vi "Write_Bypass.vi"(0 "AccelNET.lvlib:TCP.lvclass":refnum<class "TCP.lvclass">, 2 "Pelletron Bypass":T1, 3 "error in (no error)":errorcluster) -> (10 "Error Out":errorcluster)   [LabVIEW 2012, in "AccelNET.lvlib" / "TCP.lvclass"]
uses:
  TCP.lvclass
  Bypass_Control.ctl
  Useful_SubVIs.lvlib
  Useful_Controls.lvlib
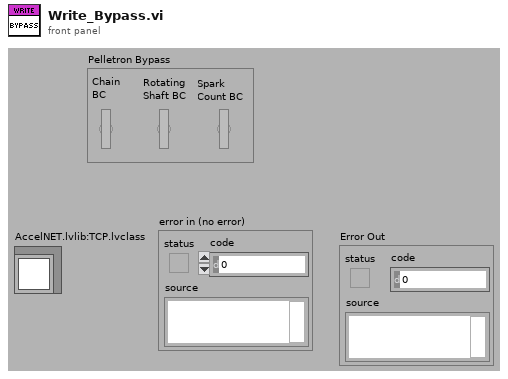
[diagram p1: front panel]
types:
  T1 = typedef "AccelNET.lvlib/Useful_Controls.lvlib/Bypass_Control.ctl" = cluster{"Chain\nBC":bool, "Rotating\nShaft BC":bool, "Spark\nCount BC":bool}
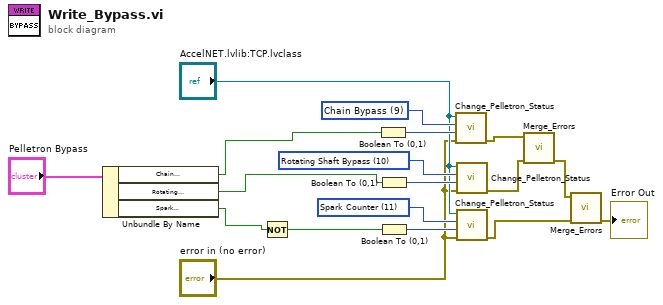
[diagram p0: block diagram]
diagram:
  w14 = u16 11 items=["GV", "Blower", "Main Power Supply", "Chain Power Supply", "Chain", "Rotating Shaft", "Power Supply Voltage", "Control Mode", "Control Mode Reference", "Chain Bypass", "Rotating Shaft Bypass", "Spark Counter", "Spark Limit", "Threshold", "Spark Counter Reset", "Ion Filament"] ("Write Selector")
  w16 = u16 10 items=["GV", "Blower", "Main Power Supply", "Chain Power Supply", "Chain", "Rotating Shaft", "Power Supply Voltage", "Control Mode", "Control Mode Reference", "Chain Bypass", "Rotating Shaft Bypass", "Spark Counter", "Spark Limit", "Threshold", "Spark Counter Reset", "Ion Filament"] ("Write Selector")
  w18 = u16 9 items=["GV", "Blower", "Main Power Supply", "Chain Power Supply", "Chain", "Rotating Shaft", "Power Supply Voltage", "Control Mode", "Control Mode Reference", "Chain Bypass", "Rotating Shaft Bypass", "Spark Counter", "Spark Limit", "Threshold", "Spark Counter Reset", "Ion Filament"] ("Write Selector")
  n1 = Unbundle By Name("Pelletron Bypass") -> ("Chain\nBC"=w4:bool, "Rotating\nShaft BC"=w3:bool, "Spark\nCount BC"=w2:bool)
  n2 = Not(x=w2) -> (.not. x?=w1:bool)
  n3 = Boolean To (0,1)(Boolean=w4) -> (0, 1=w17:i16)
  n4 = Boolean To (0,1)(Boolean=w3) -> (0, 1=w15:i16)
  n5 = Boolean To (0,1)(Boolean=w1) -> (0, 1=w13:i16)
  n6 = call "Change_Pelletron_Status.vi"("error in (no error)"="error in (no error)", "Write Value"=w17, "Write Selector"=w18, "AccelNET.lvlib:TCP.lvclass"="AccelNET.lvlib:TCP.lvclass") -> ("error out"=w10:errorcluster)  [unwired: 7 in]
  n7 = call "Change_Pelletron_Status.vi"("error in (no error)"="error in (no error)", "Write Value"=w15, "Write Selector"=w16, "AccelNET.lvlib:TCP.lvclass"="AccelNET.lvlib:TCP.lvclass") -> ("error out"=w9:errorcluster)  [unwired: 7 in]
  n8 = call "Change_Pelletron_Status.vi"("error in (no error)"="error in (no error)", "Write Value"=w13, "Write Selector"=w14, "AccelNET.lvlib:TCP.lvclass"="AccelNET.lvlib:TCP.lvclass") -> ("error out"=w8:errorcluster)  [unwired: 7 in]
  n9 = call "Merge_Errors.vi"("Error 2"=w9, "Error 1"=w10) -> ("Error Out"=w7:errorcluster)  [unwired: 9 in]
  n10 = call "Merge_Errors.vi"("Error 2"=w8, "Error 1"=w7) -> ("Error Out"=→"Error Out":errorcluster)  [unwired: 9 in]
